vi "Autosize Window.vi"(8 "error in (no error)":errorcluster, 10 "Numeric":dbl, 11 "MFC in":refnum<class "MFC.lvclass">) -> (0 "error out":errorcluster, 3 "MFC out":refnum<class "MFC.lvclass">)   [LabVIEW 2013]
uses:
  MFC.lvclass
  MFC.lvclass/MFC.ctl
  Read VI Refnum.vi
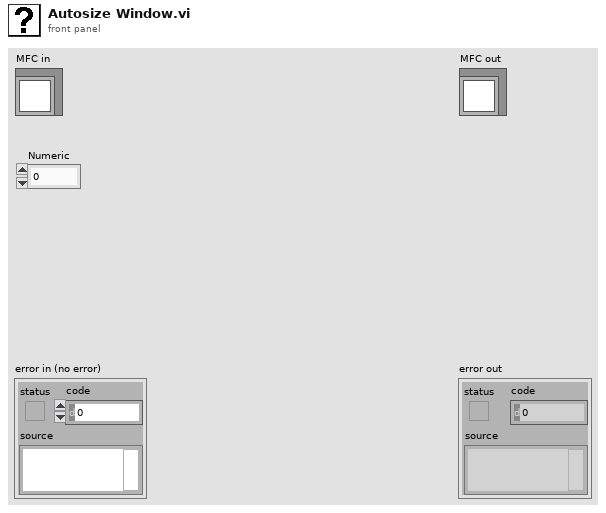
[diagram p1: front panel]
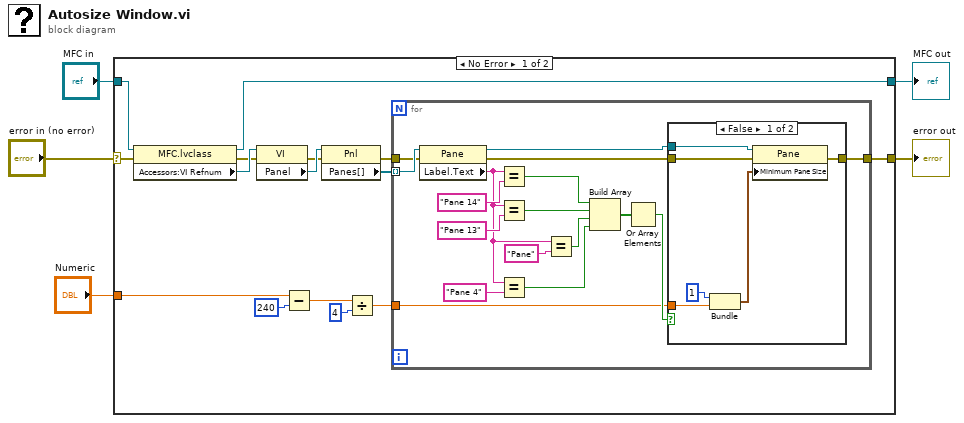
[diagram p0: block diagram]
diagram:
  n1 = case shown="No Error" "error in (no error)" {
    selector: "error in (no error)" -> [w18 w46]
    tunnel: [w8 w46] -> w4
    tunnel: [w19 w45] -> w2
    tunnel: "MFC in" -> [w20 w45]
    tunnel: "Numeric" -> [w6 _]
    frame No Error {
      n2 = property class="MFC.lvclass"(reference=w20, error in=w18) -> (reference out=w19:refnum<class "MFC.lvclass">, error out=w7:errorcluster, "Accessors:VI Refnum"=w17:refnum<vi>)
      n3 = property class="VI"(reference=w17, error in=w7) -> (error out=w15:errorcluster, "Panel"=w16:refnum<vi>)  [unwired: 1 out]
      n4 = Subtract(x=w6, y=u32 240) -> (x-y=w11:dbl)
      n5 = property class="Pnl"(reference=w16, error in=w15) -> (error out=w13:errorcluster, "Panes[]"=w14:refnum<vi>[])  [unwired: 1 out]
      n6 = Divide(x=w11, y=u32 4) -> (x/y=w9:dbl)
      n7 = for {
        tunnel: w14 -> [w37] mode=indexing
        tunnel: w13 -> [w24]
        tunnel: w9 -> [w22]
        tunnel: [w21] -> w8
        n8 = property class="Pane"(reference=w37, error in=w24) -> (reference out=w36:refnum<vi>, error out=w23:errorcluster, "Label.Text"=w31:string)
        n9 = Equal?(x=w31, y="Pane 14") -> (x = y?=w30:bool)
        n10 = Equal?(x=w31, y="Pane 13") -> (x = y?=w29:bool)
        n11 = Equal?(x=w31, y="Pane 4") -> (x = y?=w27:bool)
        n12 = Equal?(x=w31, y="Pane") -> (x = y?=w28:bool)
        n13 = Build Array(w30, w29, w28, w27) -> (w26:bool[])
        n14 = Or Array Elements(Boolean array=w26) -> (logical OR=w25:bool)
        n15 = case shown="False" w25 {
          tunnel: w36 -> [w43 _]
          tunnel: w23 -> [w42 w44]
          tunnel: w22 -> [w39 _]
          tunnel: [w38 w44] -> w21
          frame False {
            n16 = Bundle("y"=u32 1, w39) -> (w41:cluster{"y":u32, dbl})  [unwired: 1 in]
            n17 = property class="Pane"(reference=w43, error in=w42, "Minimum Pane Size"=w41) -> (error out=w38:errorcluster)  [unwired: 1 out]
          }
          frame True {
          }
        }
      }
    }
    frame Error {
    }
  }
  "error out" <- w4
  "MFC out" <- w2
